vi "Validate Credentials Remote Machine.vi"(7 "machine":string, 8 "error in (no error)":errorcluster, 10 "password":string, 11 "userName":string) -> (0 "error out":errorcluster, 3 "valid":bool)   [LabVIEW 2017, in "Windows Security.lvlib"]
doc: "Validate the credentials against a remote machine."
uses:
  Windows Security.lvlib
  System.DirectoryServices.AccountManagement
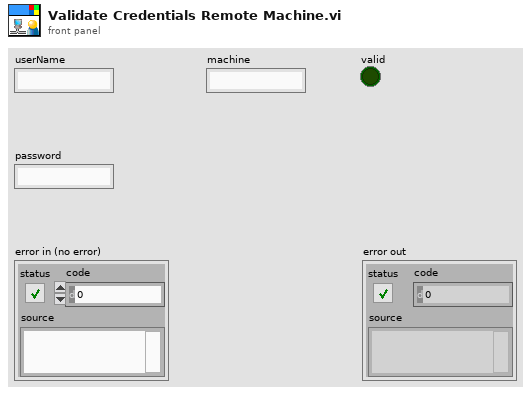
[diagram p1: front panel]
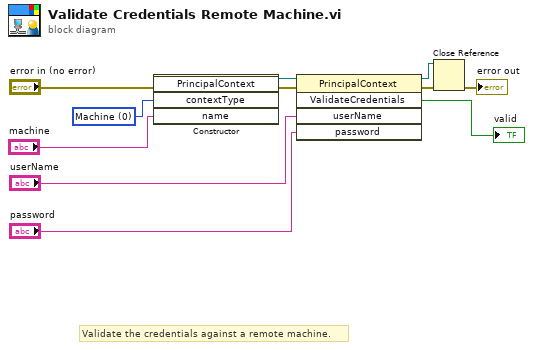
[diagram p0: block diagram]
diagram:
  w11 = 0 items=["Machine", "Domain", "ApplicationDirectory"] ("contextType")
  # "Validate the credentials against a remote machine."
  n1 = constructor class="PrincipalContext"(error in="error in (no error)", "contextType"=w11, "name"="machine") -> (reference out=w9:refnum<k24>, error out=w8:errorcluster)  [unwired: 2 in, 3 out]
  n2 = invoke class="PrincipalContext" method="ValidateCredentials"(reference=w9, error in=w8, "userName"="userName", "password"="password") -> (reference out=w6:refnum<k24>, error out=w7:errorcluster, "ValidateCredentials"=→"valid":bool)  [unwired: 1 in, 2 out]
  n3 = Close Reference(reference=w6, error in (no error)=w7) -> (error out=→"error out":errorcluster)
